vi "Idle State Update.vi"(11 "Worker Block In":T1={"Block Status"=refnum, "Command Queue"=refnum, "Status"={"Block Status"={"State"=enum."Init", "Next State"=enum."Idle", "Runs"=0, "i"=0, "Init"=FALSE, "Started"=FALSE, "Closing"=FALSE, "Step"=FALSE, "Phase"=enum."N/A", "Worker"=""}, "Error"={"status"=FALSE, "code"=0, "source"=""}}}) -> (3 "Worker Block":T1={"Block Status"=refnum, "Command Queue"=refnum, "Status"={"Block Status"={"State"=enum."Init", "Next State"=enum."Idle", "Runs"=0, "i"=0, "Init"=FALSE, "Started"=FALSE, "Closing"=FALSE, "Step"=FALSE, "Phase"=enum."N/A", "Worker"=""}, "Error"={"status"=FALSE, "code"=0, "source"=""}}})   [LabVIEW 2022 SP3, in "FlexBlocks Support.lvlib"]
uses:
  FlexBlocks Support.lvlib
  Worker Block.ctl
  Block Status with Error.ctl
  Block Status.ctl
  Block State.ctl
  Block Phase.ctl
  Block Command.ctl
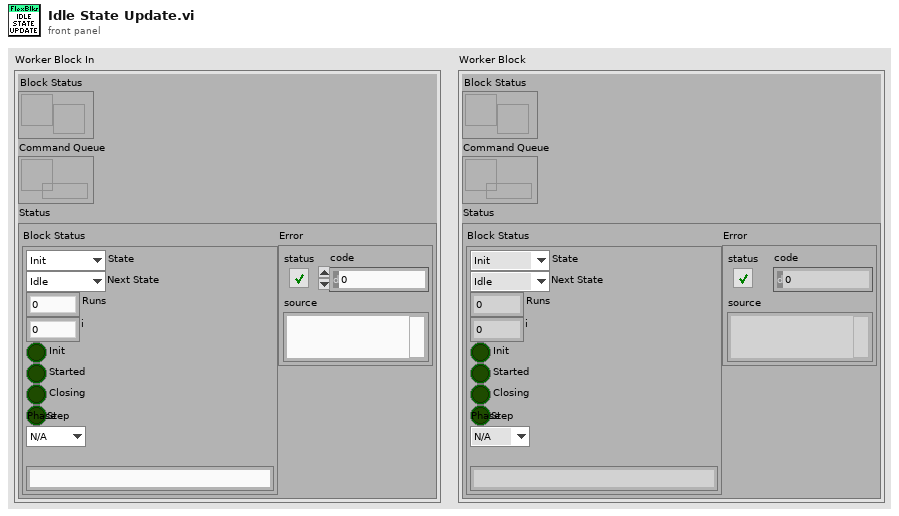
[diagram p1: front panel]
types:
  T1 = typedef "FlexBlocks Support.lvlib/Worker Block.ctl" = cluster{"Block Status":refnum<user-event>, "Command Queue":refnum<queue>, "Status":T2}
  T2 = typedef "FlexBlocks Support.lvlib/Block Status with Error.ctl" = cluster{"Block Status":T3, "Error":errorcluster}
  T3 = typedef "FlexBlocks Support.lvlib/Block Status.ctl" = cluster{"State":T4, "Next State":T4, "Runs":u32, "i":i32, "Init":bool, "Started":bool, "Closing":bool, "Step":bool, "Phase":T5, "Worker":string}
  T4 = typedef "FlexBlocks Support.lvlib/Block State.ctl" = enum16{"Idle", "Init", "Start", "Run", "Stop", "Close"}
  T5 = typedef "FlexBlocks Support.lvlib/Block Phase.ctl" = enum16{"N/A", "Read", "Work", "Write"}
  T6 = typedef "FlexBlocks Support.lvlib/Block Command.ctl" = enum16{"Close", "Init", "Step", "Run", "Pause"}
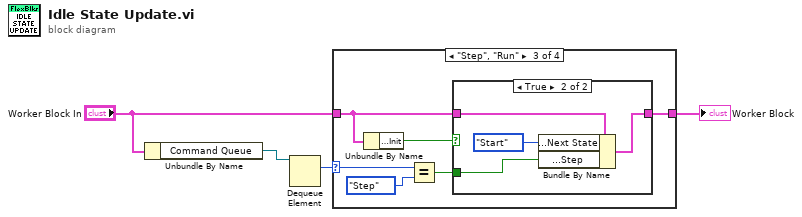
[diagram p0: block diagram]
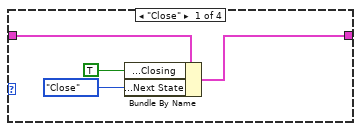
[diagram p2: hidden frame]
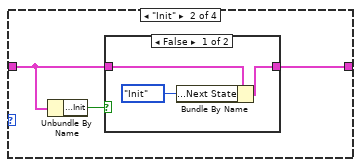
[diagram p3: hidden frame]
diagram:
  n1 = Unbundle By Name("Worker Block In") -> ("Command Queue"=w4:refnum<queue>)
  n2 = Dequeue Element(queue=w4) -> (element=w3:T6)  [unwired: 2 in, 3 out]
  n3 = case shown="\"Step\", \"Run\"" w3 {
    selector: w3 -> [_ _ w18 _]
    tunnel: "Worker Block In" -> [w8 w10 w20 w27]
    tunnel: [w5 w9 w19 w27] -> w1
    frame "Close" {
      n4 = Bundle By Name(cluster=w8, "Status.Block Status.Closing"=TRUE, "Status.Block Status.Next State"=Block_State."Close" ("Status.Block Status.State")) -> (w5:T1)
    }
    frame "Init" {
      n5 = Unbundle By Name(w10) -> ("Status.Block Status.Init"=w11:bool)
      n6 = case shown="False" w11 {
        tunnel: w10 -> [w14 w15]
        tunnel: [w12 w15] -> w9
        frame False {
          n7 = Bundle By Name(cluster=w14, "Status.Block Status.Next State"=Block_State."Init" ("Status.Block Status.State")) -> (w12:T1)
        }
        frame True {
        }
      }
    }
    frame "Step", "Run" {
      n8 = Unbundle By Name(w20) -> ("Status.Block Status.Init"=w21:bool)
      n9 = Equal?(x=w18, y=Block_Command."Step") -> (x = y?=w16:bool)
      n10 = case shown="True" w21 {
        tunnel: w20 -> [w22 w26]
        tunnel: [w22 w25] -> w19
        tunnel: w16 -> [_ w23]
        frame False {
        }
        frame True {
          n11 = Bundle By Name(cluster=w26, "Status.Block Status.Next State"=Block_State."Start" ("Status.Block Status.State"), "Status.Block Status.Step"=w23) -> (w25:T1)
        }
      }
    }
    frame "Pause" {
    }
  }
  "Worker Block" <- w1
